vi "ScalerTest1.vi"() -> ()   [LabVIEW 2009]
panel:
  out "AttGain":dbl
  in  "Att Ind":u8(knob) scale=0.0..1.0
  in  "Ib Ind":u8(knob) scale=0.0..2.0
  in  "Clip Ind":u8(knob) scale=0.0..2.0
  in  "Volt Ind Ind":u8(knob) scale=0.0..4.0
  in  "Clip Sel":i32[](array[numeric])=[7, 31, 63]
  in  "Att":i32[](array[numeric])=[0, 15]
  in  "IB_Clip":i32[](array[numeric])=[7, 31, 63]
  in  "Voltages":dbl[](array[numeric])=[0.05, 0.1, 0.2, 0.5, 0.8]
  out "V Offset4":dbl
  out "Vert Range":dbl
  out "V Offset3":dbl
  out "V Offset1":dbl
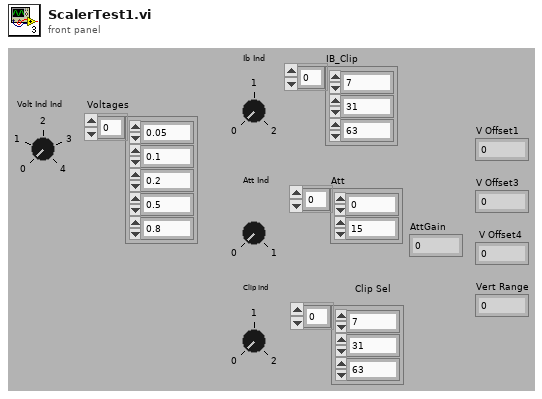
[diagram p1: front panel]
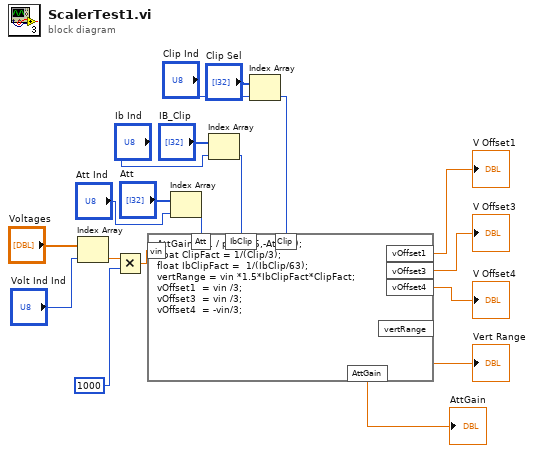
[diagram p0: block diagram]
diagram:
  n1 = Index Array(array="Voltages", index="Volt Ind Ind") -> (element=w3:dbl)
  n2 = Multiply(x=w3, y=1000) -> (x*y=w4:dbl)
  n3 = Index Array(array="Att", index="Att Ind") -> (element=w15:i32)
  n4 = Index Array(array="IB_Clip", index="Ib Ind") -> (element=w14:i32)
  n5 = Index Array(array="Clip Sel", index="Clip Ind") -> (element=w13:i32)
  n6 = formula code="AttGain = 1 / pow(1.5,-Att/10);\nfloat ClipFact = 1/(Clip/3);\nfloat IbClipFact =  1/(IbClip/63);\nvertRange = vin *1.5*IbClipFact*ClipFact;\nvOffset1  = vin /3;\nvOffset3  = vin /3;\nvOffset4  = -vin/3;"("vin"=w4, "IbClip"=w14, "Clip"=w13, "Att"=w15) -> ("vOffset1"=→"V Offset1":dbl, "vOffset3"=→"V Offset3":dbl, "vOffset4"=→"V Offset4":dbl, "vertRange"=→"Vert Range":dbl, "AttGain"=→"AttGain":dbl)
